vi "Initiate Updates.vi"(8 "error in (no error)":errorcluster, 11 "IViewModel In":refnum<class "IViewModel.lvclass">) -> (0 "error out":errorcluster, 3 "IViewModel Out":refnum<class "IViewModel.lvclass">)   [LabVIEW 2017, in "IViewModel.lvlib" / "IViewModel.lvclass"]
doc: "<License>\nCopyright © 2017 Composed Systems, LLC | All rights reserved\nwww.composed.io\n\nAuthor: Ethan Stern <ethan.stern@composed.io>\n\nThis software is provided \"AS IS\" WITHOUT WARRANTIES, either express or implied, AND IS FOR EDUCATIONAL PURPOSES ONLY.\n</License>"
uses:
  IViewModel.lvclass
  C:/Git/mva-framework/Framework/IViewable/IViewable/IViewable.lvclass
  IViewable/IViewable/IViewable.lvclass/IViewable.ctl
  IViewManager/IViewManager/IViewManager.lvclass
  IViewable/IViewable/IViewable.lvclass
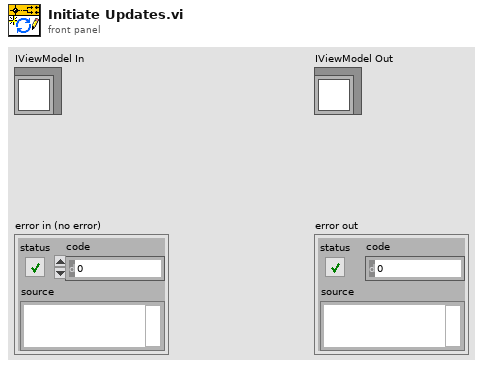
[diagram p1: front panel]
types:
  T1 = enum32{"Invalid", "Standard", "Closed", "Hidden", "Minimized", "Maximized"}
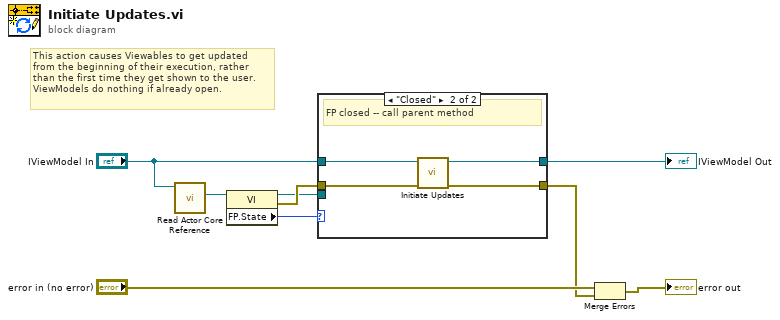
[diagram p0: block diagram]
diagram:
  # "This action causes Viewables to get updated\nfrom the beginning of their execution, rather\nthan the first time they get shown to the user.\nViewModels do nothing if already open."
  n1 = call "Read Actor Core Reference.vi"("IViewable In"="IViewModel In") -> ("Actor Core Refnum"=w4:refnum<vi>)  [unwired: 9 in, 1 out]
  n2 = property class="VI"(reference=w4) -> (reference out=w2:refnum<vi>, error out=w3:errorcluster, "FP.State"=w1:T1)  [unwired: 1 in]
  n3 = case shown="\"Closed\"" w1 {
    tunnel: "IViewModel In" -> [w11 w15]
    tunnel: [w11 w14] -> w6
    tunnel: [w10 w13] -> w5
    tunnel: w3 -> [w10 w12]
    tunnel: w2 -> [_ _]
    frame Default {
      # "FP not closed -- do nothing"
    }
    frame "Closed" {
      # "FP closed -- call parent method"
      n4 = call-parent "Initiate Updates.vi"("error in (no error)"=w12, "IViewable In"=w15) -> ("error out"=w13:errorcluster, "IViewable Out"=w14:refnum<class "IViewModel.lvclass">)  [unwired: 8 in]
    }
  }
  "IViewModel Out" <- w6
  n5 = Merge Errors("error in (no error)", w5) -> (→"error out":errorcluster)
